vi "Vision Processing.vi"(4 "error in (no error)":errorcluster) -> ()   [LabVIEW 2012]
doc: "This VI runs in parallel to other tasks. It gets images from the camera, processes them for color or shape and use that information to affect robot behavior."
uses:
  Robot Global Data.vi
  <vilib>/vision/NI_Vision_Development_Module.lvlib
panel:
  out "Original Image":T1(plugin-control)
  in  "View":bool
  in  "Area Size Limit":i32=444
  in  "Particle Count Limit":i32=10
  in  "Height of target from camera":dbl
  out "Annotated Image":T1(plugin-control)
  in  "Processing":enum32{"Color", "Intensity"}(tab)
  in  "Luminance":i32=200
  in  "Saturation":i32=50
  in  "Hue":i32(knob)=121 scale=0.0..255.0
  in  "Margins":cluster{"Hue":i32, "Sat":i32, "Lum":i32}={"Hue"=40, "Sat"=40, "Lum"=20} {"Sat" scale=0.0..40.0; "Lum" scale=0.0..40.0; "Hue" scale=0.0..40.0}
  # "This is unit-insensitive, outputs in whatever unit you feed it."
  # "Yeah, um, don't use this.\n\n[We never have, so...]"
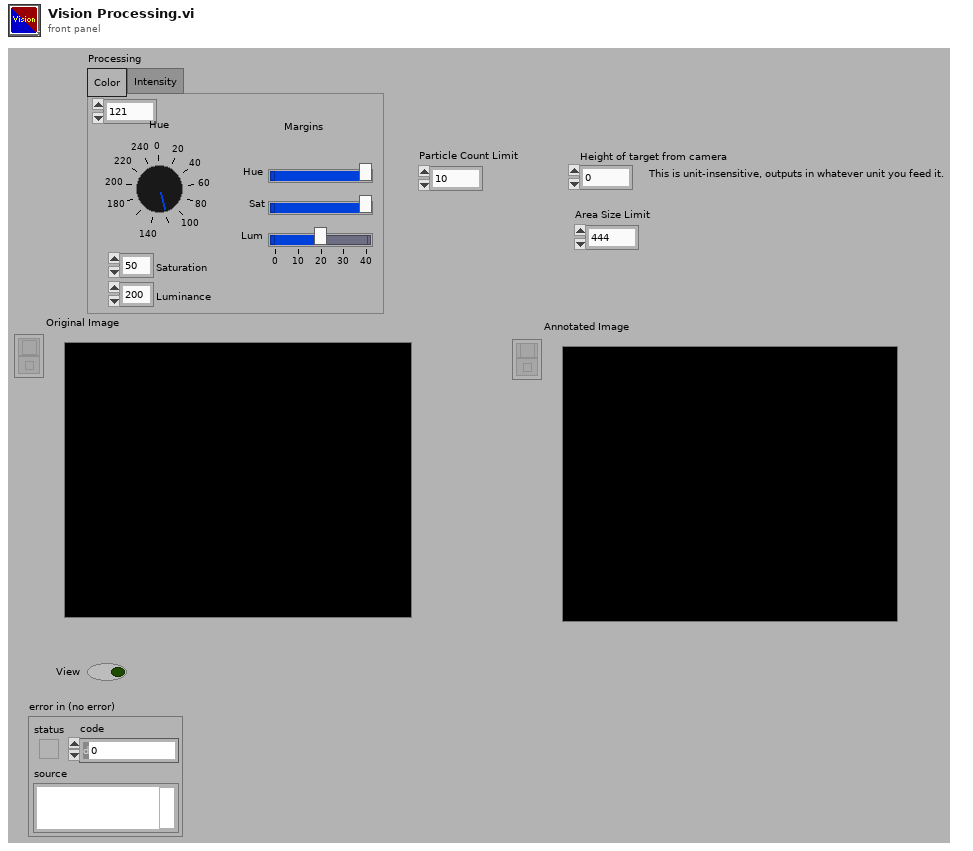
[diagram p1: front panel]
types:
  T1 = typedef "IMAQ Image.ctl" = refnum<image>
  T2 = typedef "Image Type" = u32
  T3 = typedef "WPI_CameraDevRef.ctl" = cluster{"Camera Address":string, "CameraStatus":errorcluster, "Acquire Image Notifier":refnum<notifier>}
  T4 = typedef "CameraResolutionInfo.ctl" = cluster{"X Image Resolution":i32, "Y Image Resolution":i32, "FoV X":dbl, "FoV Y":dbl, "X scale":dbl, "Y scale":dbl}
  T5 = typedef "WPI_CameraImageSize.ctl" = enum16{"640x480", "320x240", "160x120"}
  T6 = cluster{cluster{"Left":dbl, "Top":dbl, "Right":dbl, "Bottom":dbl}, "Scores":dbl[], cluster{"Long":dbl, "Short":dbl}}[]
  T7 = cluster{"Left":dbl, "Top":dbl, "Right":dbl, "Bottom":dbl}
  T8 = cluster{"Left":dbl, "Top":dbl, "Right":dbl, "Bottom":dbl}[]
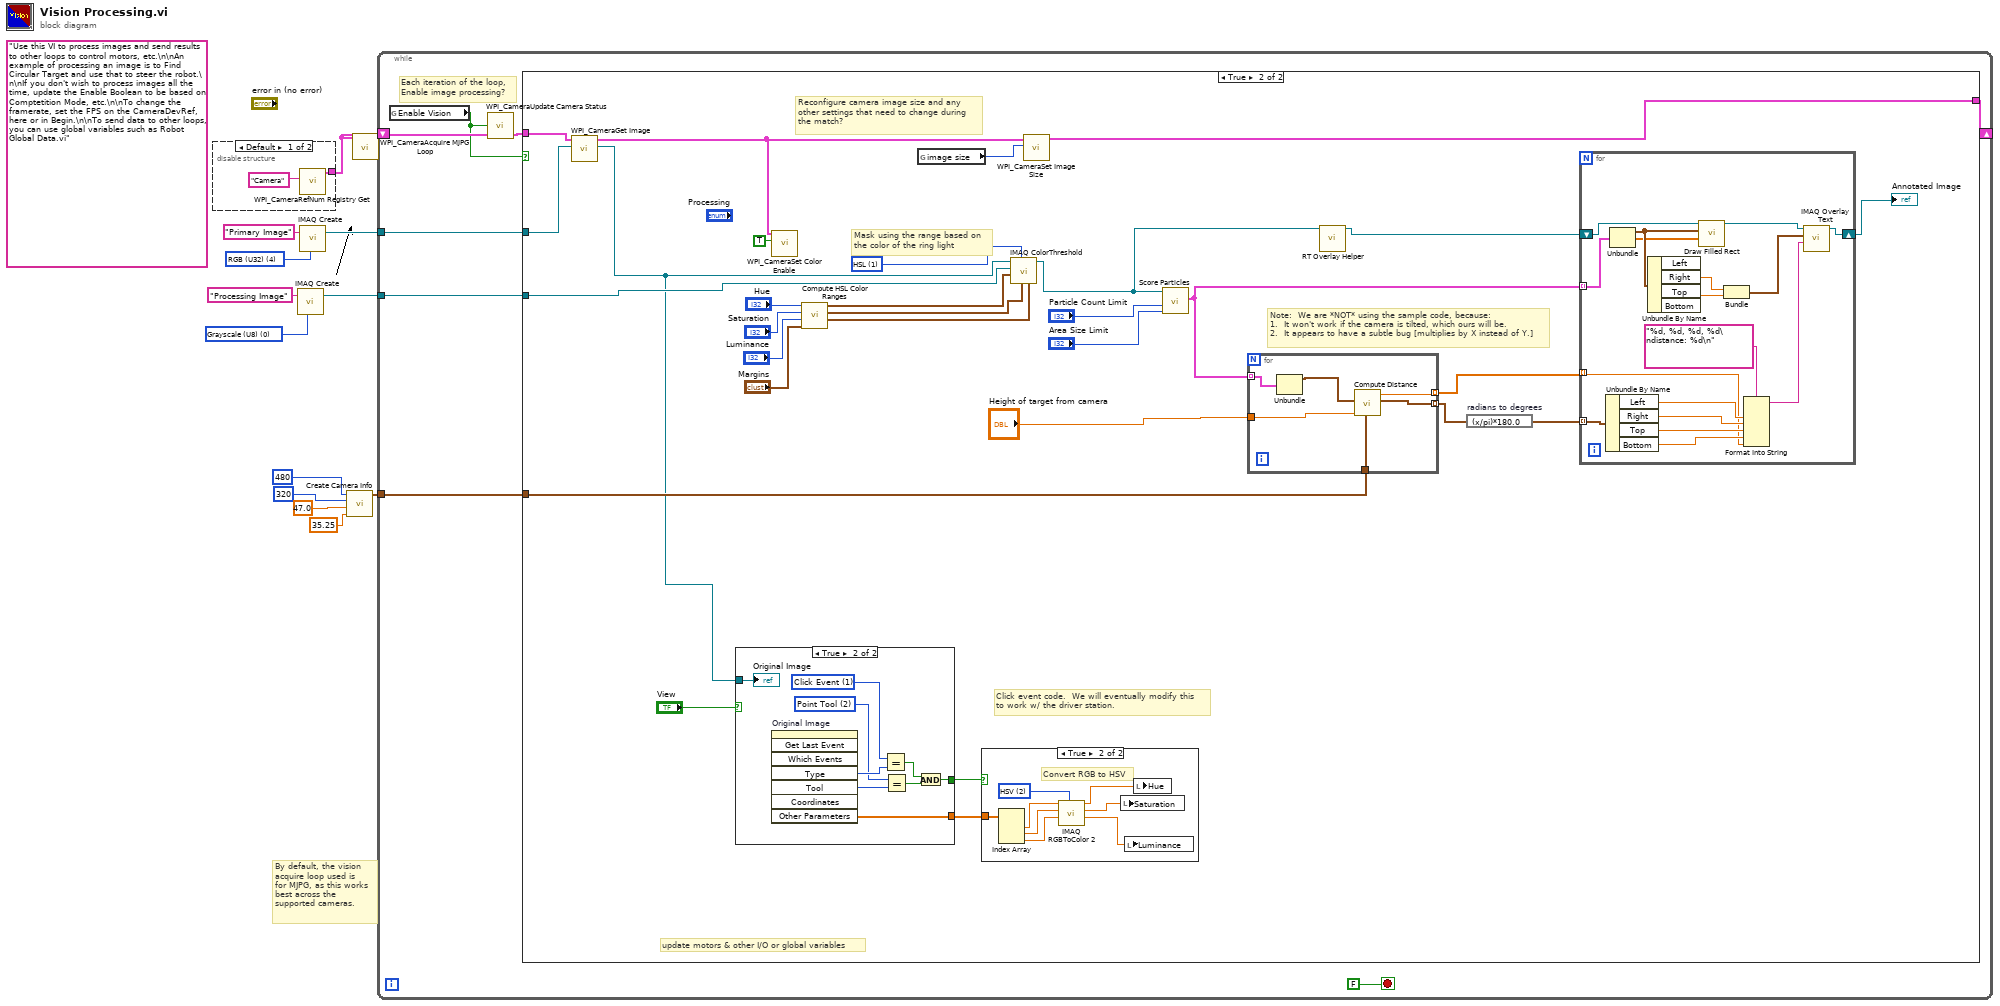
[diagram p0: block diagram]
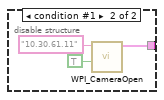
[diagram p2: hidden frame]
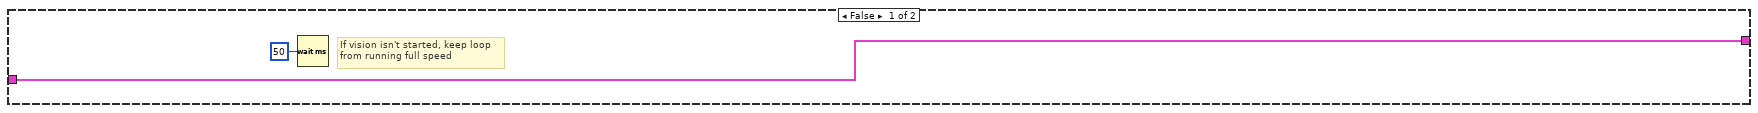
[diagram p3: hidden frame]
diagram:
  w4 = T2 0 items=["Grayscale (U8)", "Grayscale (I16)", "Grayscale (SGL)", "Complex (CSG)", "RGB (U32)", "HSL (U32)", "RGB (U64)"] ("Image Type")
  w6 = T2 4 items=["Grayscale (U8)", "Grayscale (I16)", "Grayscale (SGL)", "Complex (CSG)", "RGB (U32)", "HSL (U32)", "RGB (U64)"] ("Image Type")
  (unwired) "Use this VI to process images and send results to other loops to control motors, etc.\n\nAn example of processing an image is to Find Circular Target and use that to steer the robot.\n\nIf you don't wish to process images all the time, update the Enable Boolean to be based on Comptetition Mode, etc.\n\nTo change the framerate, set the FPS on the CameraDevRef, here or in Begin.\n\nTo send data to other loops, you can use global variables such as Robot Global Data.vi"
  # "By default, the vision\nacquire loop used is\nfor MJPG, as this works\nbest across the\nsupported cameras."
  n1 = disable-structure shown="Default" {
    disable-tunnel: [w13 w16] -> w7
    frame condition #0 (active) {
      n2 = call <vilib>:"WPI_CameraRefNum Registry Get.vi"("refnum name"="Camera") -> ("CameraDevRef"=w13:T3)  [unwired: 1 in, 9 out]
    }
    frame condition #1 {
      n3 = call <vilib>:"WPI_CameraOpen.vi"(9:TRUE ("Disallow Simulation"), "Camera Address"="10.30.61.11") -> ("CameraDevRef"=w16:T3)  [unwired: 8 in, 1 out]
    }
  }
  n4 = call "IMAQ Create"("Image Name"="Processing Image", "Image Type"=w4) -> ("New Image"=w11:T1)  [unwired: 2 in, 2 out]
  n5 = call "IMAQ Create"("Image Name"="Primary Image", "Image Type"=w6) -> ("New Image"=w12:T1)  [unwired: 2 in, 2 out]
  n6 = call "Create Camera Info.vi"("FoV Y"=35.25 ("FoV X"), "FoV X"=47.0, "Y Image Resolution"=320, "X Image Resolution"=480) -> ("Camera Info"=w10:T4)  [unwired: 7 in]
  n7 = call <vilib>:"WPI_CameraAcquire MJPG Loop.vi"("CameraDevRef"=w7) -> ()  [unwired: 11 in]
  n8 = while {
    shift-right: [w24] -> _
    shift-left: w7 -> [w22]
    tunnel: w12 -> [w23]
    tunnel: w11 -> [w20]
    tunnel: w10 -> [w19]
    stop <- FALSE stop-if-true
    # "Each iteration of the loop,\nEnable image processing?"
    n9 = global read "Robot Global Data.vi" "Enable Vision"() -> (w18:bool)
    n10 = call <vilib>:"WPI_CameraUpdate Camera Status.vi"("CameraDevRef In"=w22, "Enable Vision"=w18) -> ("CameraDevRef Out"=w21:T3)  [unwired: 3 in]
    n11 = case shown="True" w18 {
      tunnel: w23 -> [_ w56]
      tunnel: [w27 w57] -> w24
      tunnel: w21 -> [w27 w54]
      tunnel: w20 -> [_ w52]
      tunnel: w19 -> [_ w51]
      frame False {
        # "If vision isn't started, keep loop\nfrom running full speed"
        n12 = Wait (ms)(milliseconds to wait=u32 50) -> ()  [unwired: 1 out]
      }
      frame True {
        w41 = u16 1 items=["RGB", "HSL", "HSV", "HSI"] ("Color Mode")
        # "Note:  We are *NOT* using the sample code, because:\n1.  It won't work if the camera is tilted, which ours will be.\n2.  It appears to have a subtle bug [multiplies by X instead of Y.]"
        # "Mask using the range based on\nthe color of the ring light"
        # "Click event code.  We will eventually modify this\nto work w/ the driver station."
        # "update motors & other I/O or global variables"
        # "Reconfigure camera image size and any\nother settings that need to change during\nthe match?"
        n13 = call <vilib>:"WPI_CameraGet Image.vi"("Image"=w56, "CameraDevRef"=w54) -> ("Image Out"=w44:T1, "CameraDevRef Out"=w53:T3)  [unwired: 1 in, 7 out]
        n14 = case shown="True" "View" {
          tunnel: [_ w87] -> w47
          tunnel: [_ w84] -> w46
          tunnel: w44 -> [_ w83]
          frame False {
          }
          frame True {
            w85 = 2 items=["None", "Selection Tool", "Point Tool", "Line Tool", "Rectangle Tool", "Oval Tool", "Polygon Tool", "ClosedFreehandTool", "Annulus Tool", "Rotated Rectangle Tool", "Zoom Tool", "Pan Tool", "Polyline Tool", "Freehand Tool"] ("Tool")
            w86 = 1 items=["No Event"=0, "Click Event"=1, "Draw Event"=2, "Size Event"=4, "Scroll Event"=5, "Double Click Event"=8] ("Type")
            n15 = invoke on="Original Image" class="ImageControl" method="Get Last Event"() -> ("Type"=w88:i32, "Tool"=w91:i32, "Other Parameters"=w84:sgl[])  [unwired: 8 in, 5 out]
            n16 = Equal?(x=w86, y=w88) -> (x = y?=w89:bool)
            n17 = Equal?(x=w85, y=w91) -> (x = y?=w90:bool)
            n18 = And(x=w89, y=w90) -> (x .and. y?=w87:bool)
            "Original Image" <- w83
          }
        }
        n19 = call <vilib>:"WPI_CameraSet Color Enable.vi"("Color Enabled"=TRUE, "CameraDevRef"=w53) -> ()  [unwired: 8 in, 2 out]
        n20 = call "Compute HSL Color Ranges.vi"("Margins"="Margins", "Luminance"="Luminance", "Saturation"="Saturation", "Hue"="Hue") -> ("Lum Range"=w38:cluster{i32, i32}, "Sat Range"=w39:cluster{i32, i32}, "Hue Range"=w40:cluster{i32, i32})  [unwired: 5 in]
        n21 = global read "Robot Global Data.vi" "image size"() -> (w55:T5)
        n22 = case shown="True" w47 {
          tunnel: w46 -> [_ w82]
          frame False {
          }
          frame True {
            w81 = u16 2 items=["RGB", "HSL", "HSV", "HSI", "CIE L*a*b*", "CIE XYZ"] ("Color Mode")
            # "Convert RGB to HSV"
            n23 = Index Array(array=w82) -> (element #1=w80:sgl, element #2=w79:sgl, element #3=w78:sgl)  [unwired: 3 in]
            n24 = call "IMAQ RGBToColor 2"("Color Mode"=w81, "Blue value"=w78, "Green value"=w79, "Red value"=w80) -> ("Blue or Luma or Val or Inten or Z or b*value"=w75:dbl, "Green or Sat or Y or a* value"=w76:dbl, "Red or Hue or X or L* value"=w77:dbl)  [unwired: 4 in, 1 out]
            n25 = local write "Saturation"(w76) -> ()
            n26 = local write "Luminance"(w75) -> ()
            n27 = local write "Hue"(w77) -> ()
          }
        }
        n28 = call "IMAQ ColorThreshold"("Blue or Luma or Val or Inten Range"=w38, "Green or Sat Range"=w39, "Color Mode"=w41, "Red or Hue Range"=w40, "Image Dst"=w52, "Image Src"=w44) -> ("Image Dst Out"=w32:T1)  [unwired: 4 in, 1 out]
        n29 = call <vilib>:"WPI_CameraSet Image Size.vi"("Image Size"=w55, "CameraDevRef"=w53) -> ("CameraDevRef Out"=w57:T3)  [unwired: 1 in, 8 out]
        n30 = call "Score Particles.vi"("Area Size Limit"="Area Size Limit", "Particle Count Limit"="Particle Count Limit", "Image Refnum in"=w32) -> ("Scored Particle Info"=w29:T6)  [unwired: 7 in, 1 out]
        n31 = for {
          tunnel: w29 -> [w93] mode=indexing
          tunnel: [w97] -> w50 mode=indexing
          tunnel: [w96] -> w31 mode=indexing
          tunnel: w51 -> [w95]
          tunnel: "Height of target from camera" -> [w94]
          n32 = Unbundle(w93) -> (w92:T7)  [unwired: 2 out]
          n33 = call "Compute Distance.vi"("Camera Info"=w95, "Height from camera of target"=w94, "Bounding Box"=w92) -> ("Bounding Box (Rad)"=w96:T7, "Distance to target [in 2-space]"=w97:dbl)  [unwired: 7 in]
        }
        n34 = call "RT Overlay Helper.vi"("Refnum in"=w32) -> ("Refnum out"=w28:T1)  [unwired: 10 in]
        n35 = expression code="(x/pi)*180.0" "radians to degrees"(w31) -> (w30:T8)
        n36 = for {
          tunnel: w50 -> [w59] mode=indexing
          tunnel: w30 -> [w74] mode=indexing
          shift-right: [w66] -> w49
          shift-left: w28 -> [w62]
          tunnel: w29 -> [w65] mode=indexing
          n37 = Unbundle By Name(w74) -> ("Left"=w72:dbl, "Right"=w68:dbl, "Top"=w70:dbl, "Bottom"=w69:dbl)
          n38 = Unbundle(w65) -> (w60:T7, "Scores"=w58:dbl[])  [unwired: 1 out]
          n39 = Unbundle By Name(w60) -> ("Right"=w63:dbl, "Bottom"=w64:dbl)  [unwired: 2 out]
          n40 = call "Draw Filled Rect.vi"("Scores"=w58, "Bounding Box"=w60, "image in"=w62) -> ("image out"=w61:T1)  [unwired: 8 in]
          n41 = Bundle("Right"=w63, "Bottom"=w64) -> (w67:cluster{"Right":dbl, "Bottom":dbl})  [unwired: 1 in]
          n42 = Format Into String(format string="%d, %d, %d, %d\ndistance: %d\n", w72, w68, w70, w69, w59) -> (resulting string=w71:string)  [unwired: 2 in, 1 out]
          n43 = call "IMAQ Overlay Text"("String"=w71, "Origin"=w67, "Image"=w61) -> ("Image Out"=w66:T1)  [unwired: 7 in, 1 out]
        }
        "Annotated Image" <- w49
      }
    }
  }
